vi "TestShiftRegister.vi"() -> ()   [LabVIEW 2013]
panel:
  in  "Boolean":bool
  in  "Numeric":dbl
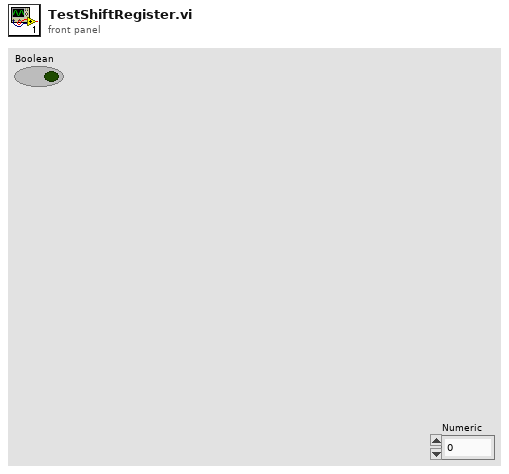
[diagram p1: front panel]
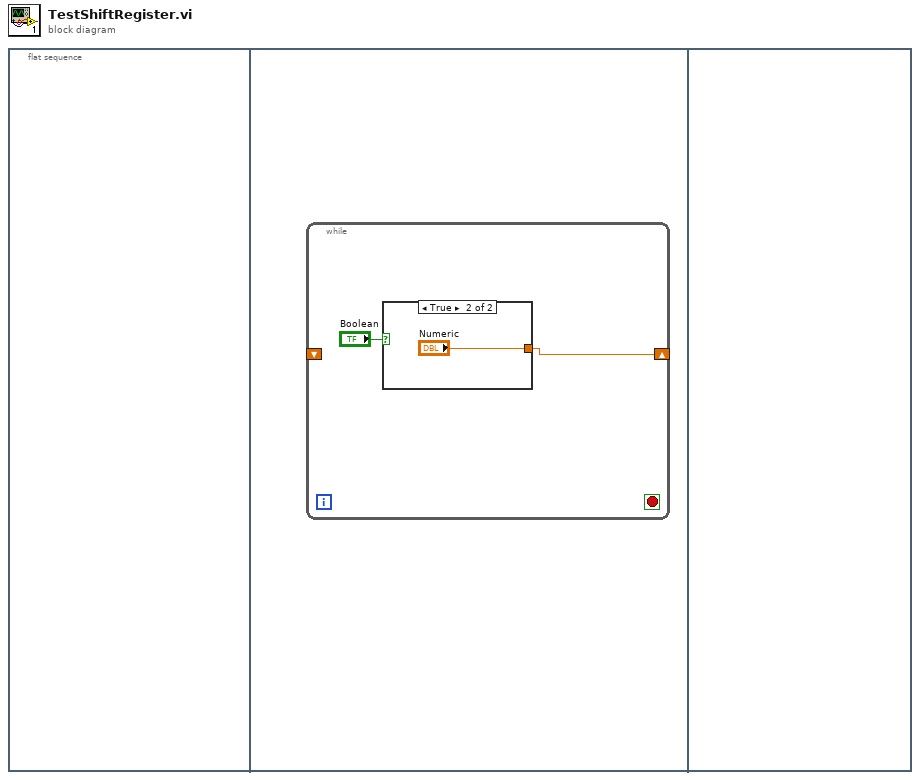
[diagram p0: block diagram]
diagram:
  n1 = flat-sequence {
    frame #0 {
    }
    frame #1 {
      n2 = while {
        shift-right: [w2] -> _
        shift-left: _ -> [_]
        stop <- _ stop-if-true
        n3 = case shown="True" "Boolean" {
          tunnel: [_ "Numeric"] -> w2
          frame False {
          }
          frame True {
          }
        }
      }
    }
    frame #2 {
    }
  }
